vi "Load Per-Site Ref Mic Sensitivity to DAQmx AI.vi"(0 "Semiconductor Module Context":T1, 11 "error in (no error)":errorcluster) -> (15 "error out":errorcluster)   [LabVIEW 2020]
uses:
  <vilib>/NI_TestStand_SemiconductorModule/NI_TestStand_Semiconductor_Module.lvlibp/PinMap/General/SemiconductorModuleContext.ctl
  03587b97-7653-4438-994b-86e0acd3bf46.vi
  03587b97-7653-4438-994b-86e0acd3bf46.vi/d77f928d-23e2-406a-91ff-9a8ae93f4cc2.vi
  <vilib>/NI_TestStand_SemiconductorModule/NI_TestStand_Semiconductor_Module.lvlibp
  <resource>/objmgr/daqmx.rc
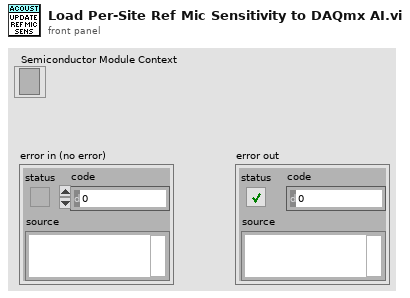
[diagram p1: front panel]
types:
  T1 = typedef "NI_TestStand_Semiconductor_Module.lvlibp/SemiconductorModuleContext.ctl" = refnum<k7>
  T2 = typedef "TSM DAQmx Multi-Task.ctl" = cluster{"Pin Query Context":refnum<class "MultiplePinMultipleSessionQueryContext.lvclass">, "SSC":T3[], "Site Numbers":i32[], "Pins":tag[]}
  T3 = typedef "SSC DAQmx.ctl" = cluster{"DAQmx Task ":refnum<k21>, "Channels":string, "Channel Lists":string}
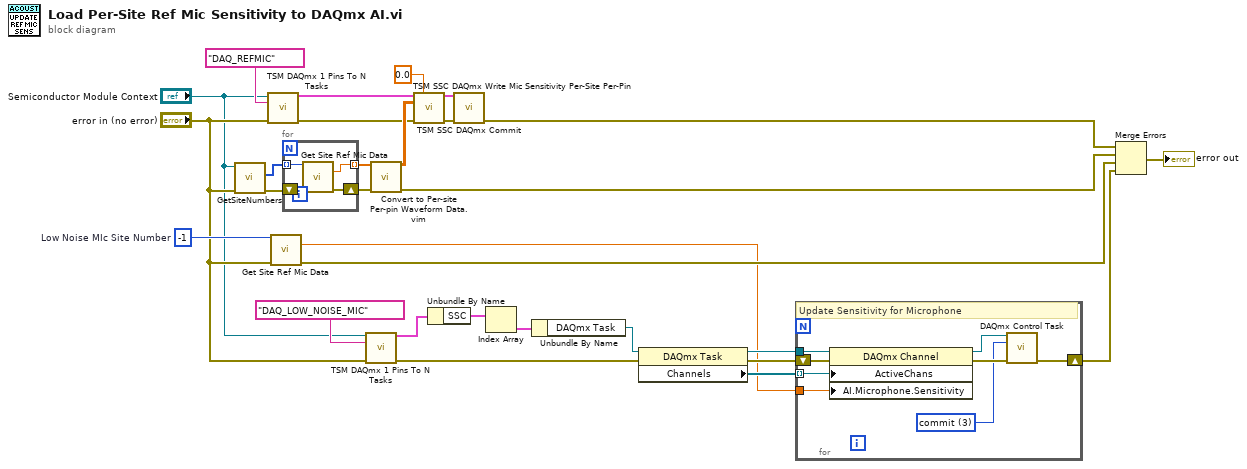
[diagram p0: block diagram]
diagram:
  w19 = -1  # Low Noise MIc Site Number
  n1 = call <vilib>:"GetSiteNumbers.vi"("error in (no error)"="error in (no error)", "Semiconductor Module Context"="Semiconductor Module Context") -> ("error out"=w14:errorcluster, "Site Numbers"=w13:i32[])  [unwired: 6 in, 2 out]
  n2 = call "TSM DAQmx 1 Pins To N Tasks.vi"("TSM context"="Semiconductor Module Context", "Pins"=tag "DAQ_REFMIC", "error in"="error in (no error)") -> ("DAQ TSM Out"=w25:T2, "error out"=w26:errorcluster)  [unwired: 11 in]
  n3 = call "Get Site Ref Mic Data.vi"("Site Number"=w19, "error in (no error)"="error in (no error)") -> ("Ref Mic Sensitivity (mV/Pa)"=w1:dbl, "error out"=w17:errorcluster)  [unwired: 10 in, 2 out]
  n4 = for {
    tunnel: [w29] -> w16 mode=indexing
    shift-right: [w32] -> w15
    shift-left: w14 -> [w31]
    tunnel: w13 -> [w30] mode=indexing
    n5 = call "Get Site Ref Mic Data.vi"("Site Number"=w30, "error in (no error)"=w31) -> ("Ref Mic Sensitivity (mV/Pa)"=w29:dbl, "error out"=w32:errorcluster)  [unwired: 10 in, 2 out]
  }
  n6 = call "TSM DAQmx 1 Pins To N Tasks.vi"("TSM context"="Semiconductor Module Context", "Pins"=tag "DAQ_LOW_NOISE_MIC", "error in"="error in (no error)") -> ("DAQ TSM Out"=w5:T2, "error out"=w7:errorcluster)  [unwired: 11 in]
  n7 = call "Convert to Per-site Per-pin Waveform Data.vim"("Waveform In"=w16) -> ("Per Site Per Pin Waveform Out"=w27:dbl[][])  [unwired: 14 in]
  n8 = call "TSM SSC DAQmx Write Mic Sensitivity Per-Site Per-Pin.vi"("DAQ TSM in"=w25, "Idle Channel Value (0)"=0.0, "Per-Site Per-Pin Mic Sensitivity in"=w27, "error in"=w26) -> ("DAQ TSM Out"=w22:T2, "error out"=w23:errorcluster)  [unwired: 10 in]
  n9 = Unbundle By Name(w5) -> ("SSC"=w4:T3[])
  n10 = call "TSM SSC DAQmx Commit.vi"("TSM DAQmx In"=w22, "error in (no error)"=w23) -> ("error out"=w21:errorcluster)  [unwired: 12 in, 1 out]
  n11 = Index Array(array=w4) -> (element=w3:T3)  [unwired: 1 in]
  n12 = Unbundle By Name(w3) -> ("DAQmx Task"=w2:refnum<k21>)
  n13 = property class="DAQmx Task"(reference=w2, error in=w7) -> (reference out=w9:refnum<k21>, error out=w10:errorcluster, "Channels"=w8:refnum<k21>[])
  n14 = for {
    tunnel: w9 -> [w33]
    tunnel: w8 -> [w40] mode=indexing
    tunnel: w1 -> [w35]
    shift-right: [w38] -> w6
    shift-left: w10 -> [w34]
    w36 = 3 items=["verify"=2, "reserve"=4, "commit"=3, "unreserve"=5, "abort"=6] ("action")
    # "Update Sensitivity for Microphone"
    n15 = property class="DAQmx Channel"(reference=w33, error in=w34, "ActiveChans"=w40, "AI.Microphone.Sensitivity"=w35) -> (reference out=w37:refnum<k21>, error out=w39:errorcluster)
    n16 = call <vilib>:"DAQmx Control Task.vi"("task/channels in"=w37, "action"=w36, "error in"=w39) -> ("error out"=w38:errorcluster)  [unwired: 11 in, 1 out]
  }
  n17 = Merge Errors(w21, w15, w17, w6) -> (→"error out":errorcluster)
